vi "Asylum_Driver_InitializeLithographyObject.vi"(4 "Abort Notifier":refnum<notifier>, 6 "Z Move Setpoint":dbl format="%#_13g", 7 "Z Write Setpoint":dbl format="%#_13g", 8 "error in (no error)":errorcluster, 9 "Offsets":cluster{"X":dbl, "Y":dbl}, 10 "Pattern Data":T2={"Name"="", "Litho"=[], "Set Resistance"=enum."1G ohm", "Meta"=variant}, 11 "Application":refnum<k7>) -> (0 "error out":errorcluster, 3 "Application":refnum<k7>)   [LabVIEW 2019]
uses:
  <userlib>/LevyLab/Relay Box/Typedefs/Resistor--enum.ctl
  <userlib>/LevyLab/Relay Box/Relay-Box.lvclass
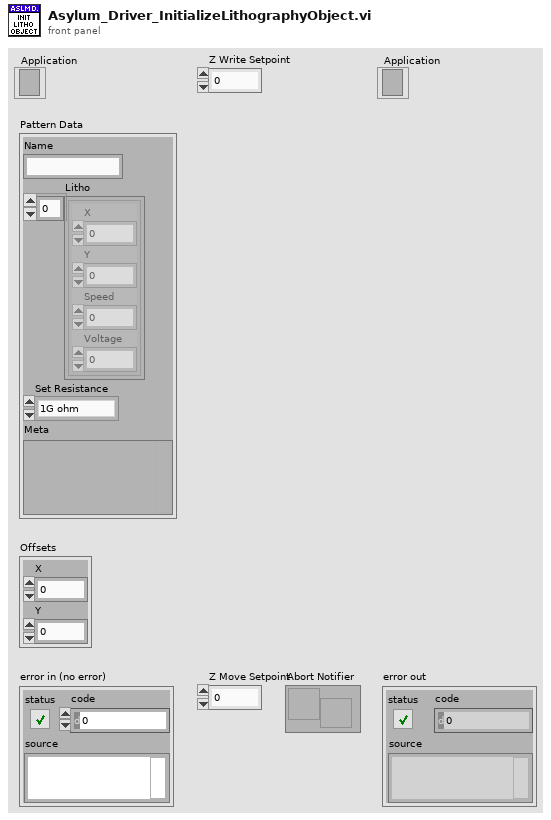
[diagram p1: front panel]
types:
  T1 = typedef "Relay-Box.lvclass/Resistor--enum.ctl" = enum16{"open", "discharge tip", "0 ohms", "100k ohm", "10M ohm", "1G ohm"}
  T2 = cluster{"Name":string, "Litho":cluster{"X":dbl, "Y":dbl, "Speed":dbl, "Voltage":dbl}[], "Set Resistance":T1, "Meta":variant}
  T3 = cluster{"X":dbl, "Y":dbl, "Speed":dbl, "Voltage":dbl}[]
  T4 = cluster{"X":dbl, "Y":dbl, "Speed":dbl, "Voltage":dbl}
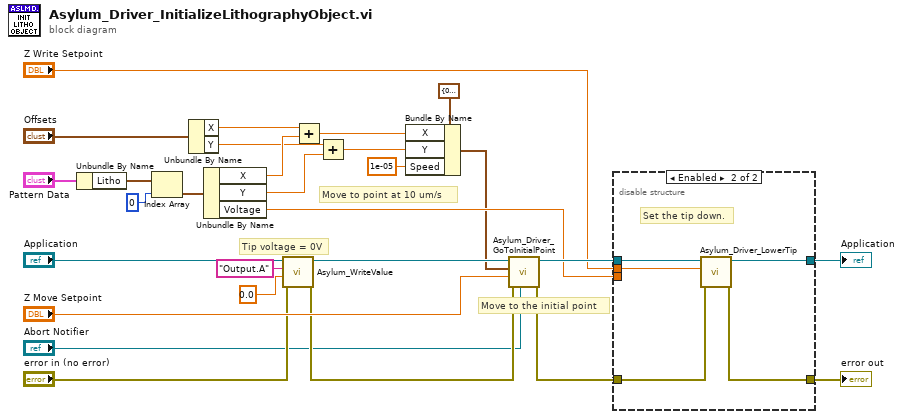
[diagram p0: block diagram]
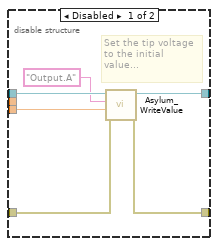
[diagram p2: hidden frame]
diagram:
  # "Move to point at 10 um/s"
  # "Move to the initial point"
  # "Tip voltage = 0V"
  n1 = Unbundle By Name("Pattern Data") -> ("Litho"=w22:T3)
  n2 = Index Array(array=w22, index=0) -> (element=w20:T4)
  n3 = Unbundle By Name("Offsets") -> ("X"=w24:dbl, "Y"=w23:dbl)
  n4 = Unbundle By Name(w20) -> ("X"=w26:dbl, "Y"=w25:dbl, "Voltage"=w5:dbl)
  n5 = call <userlib>:"Asylum_WriteValue.vi"("error in (no error)"="error in (no error)", "value"=0.0, "parameterName"="Output.A", "Application"="Application") -> ("error out"=w10:errorcluster, "Application"=w13:refnum<k7>)  [unwired: 6 in]
  n6 = Add(x=w24, y=w26) -> (x+y=w16:dbl)
  n7 = Add(x=w23, y=w25) -> (x+y=w15:dbl)
  n8 = Bundle By Name(cluster=cluster{"X":dbl, "Y":dbl, "Speed":dbl} {"X"=0.0, "Y"=0.0, "Speed"=0.0} ("Coordinate"), "X"=w16, "Y"=w15, "Speed"=1e-05) -> (w2:cluster{"X":dbl, "Y":dbl, "Speed":dbl})
  n9 = call "Asylum_Driver_GoToInitialPoint.vi"("Abort Notifier"="Abort Notifier", "error in (no error)"=w10, "Z Setpoint"="Z Move Setpoint", "Coordinate"=w2, "Application"=w13) -> ("error out"=w7:errorcluster, "Application"=w9:refnum<k7>)  [unwired: 5 in]
  n10 = disable-structure shown="Enabled" {
    disable-tunnel: w9 -> [w34 w38]
    disable-tunnel: [w33 w39] -> w8
    disable-tunnel: w7 -> [w32 w35]
    disable-tunnel: [w31 w36] -> w6
    disable-tunnel: w5 -> [w29 _]
    disable-tunnel: "Z Write Setpoint" -> [_ w37]
    frame Disabled {
      # "Set the tip voltage to the initial value..."
      n11 = call <userlib>:"Asylum_WriteValue.vi"("error in (no error)"=w32, "value"=w29, "parameterName"="Output.A", "Application"=w34) -> ("error out"=w31:errorcluster, "Application"=w33:refnum<k7>)  [unwired: 6 in]
    }
    frame Enabled {
      # "Set the tip down."
      n12 = call "Asylum_Driver_LowerTip.vi"("error in (no error)"=w35, "Z Setpoint"=w37, "Application"=w38) -> ("error out"=w36:errorcluster, "Application"=w39:refnum<k7>)  [unwired: 7 in]
    }
  }
  "Application" <- w8
  "error out" <- w6
